vi "Read ExpiresIn.vi"(8 "error in (no error)":errorcluster, 11 "Oauth2 in":refnum<class "Oauth2.lvclass">) -> (0 "error out":errorcluster, 2 "Expires In":u32, 3 "Oauth2 out":refnum<class "Oauth2.lvclass">)   [LabVIEW 2020, in "Oauth2.lvclass"]
uses:
  Oauth2.lvclass
  Oauth2.lvclass/Oauth2.ctl
  OAuthToken/OAuth2 Token Element -- enum.ctl
  OAuthToken/OAuthAccessToken.lvclass
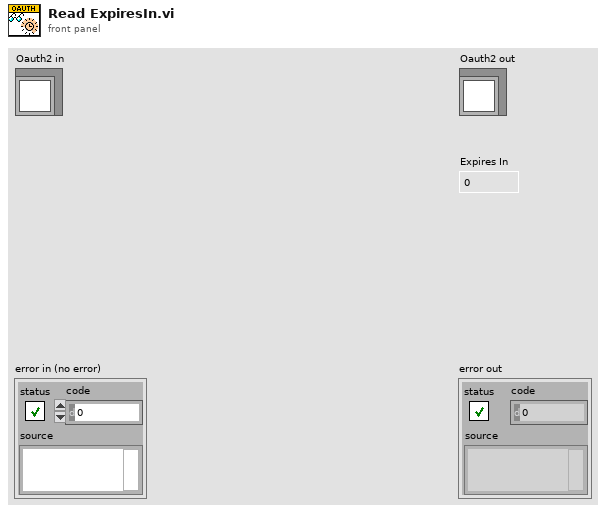
[diagram p1: front panel]
types:
  T1 = typedef "OAuthAccessToken.lvclass/OAuth2 Token Element -- enum.ctl" = enum16{"client_id", "client_secret", "response_type", "scope", "redirect_uri", "error", "error_description", "error_uri", "grant_type", "code", "access_token", "token_type", "expires_in", "username", "password", "refresh_token", "code_challenge", "code_challenge_method", "reverse_proxy_uri", "endpoint element"}
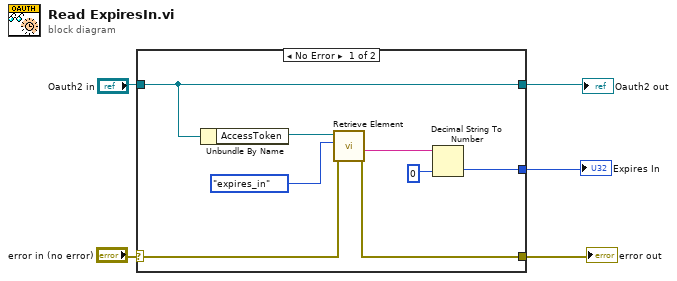
[diagram p0: block diagram]
diagram:
  n1 = case shown="No Error" "error in (no error)" {
    selector: "error in (no error)" -> [w10 w14]
    tunnel: [w9 w14] -> w3
    tunnel: [w13 w15] -> w4
    tunnel: "Oauth2 in" -> [w13 w15]
    tunnel: [w7 _] -> w1
    frame No Error {
      n2 = Unbundle By Name(w13) -> ("AccessToken"=w12:refnum<class "OAuthAccessToken.lvclass">)
      n3 = call "Retrieve Element.vi"("error in (no error)"=w10, "Token element"=OAuth2_Token_Element_--_enum."expires_in", "OAuthAccessToken in"=w12) -> ("error out"=w9:errorcluster, "Value"=w8:string)  [unwired: 4 in, 3 out]
      n4 = Decimal String To Number(string=w8, default (0L)=u32 0 ("Expires In")) -> (number=w7:u32)  [unwired: 1 in, 1 out]
    }
    frame Error {
    }
  }
  "error out" <- w3
  "Oauth2 out" <- w4
  "Expires In" <- w1
